vi "Send FindInstruments.vi"(7 "Message Priority (Normal)":T3=enum."Normal", 8 "error in (no error)":errorcluster, 10 "InstrumentData":T1, 11 "Message Enqueuer":refnum<class "Message Enqueuer.lvclass">) -> (0 "error out":errorcluster, 3 "Message Enqueuer out":refnum<class "Message Enqueuer.lvclass">)   [LabVIEW 2023, in "ZWO_ASI.lvlib" / "FindInstruments Msg.lvclass"]
doc: "This VI sends the message to an actor."
uses:
  FindInstruments Msg.lvclass
  FindInstruments Msg.lvclass/FindInstruments Msg.ctl
  <vilib>/ActorFramework/Message Enqueuer/Message Enqueuer.lvclass
  Applications/National Instruments/LabVIEW 2023 64-bit/vi.lib/ActorFramework/Message/Message.lvclass
  Users/alexandrosspiliotis/Documents/LV_DAQ_Project/ConcreteClasses/ConcreteInstrumentClasses/CameraClasses/ZWO_ASI_LV/ZWO_ASI Messages/FindInstruments Msg/FindInstruments Msg.lvclass
  <vilib>/ActorFramework/Message Enqueuer/Message Priority.ctl
  typedefs/instrumentType.ctl
  typedefs/typedefs.lvlib
  typedefs/InstrumentData.ctl
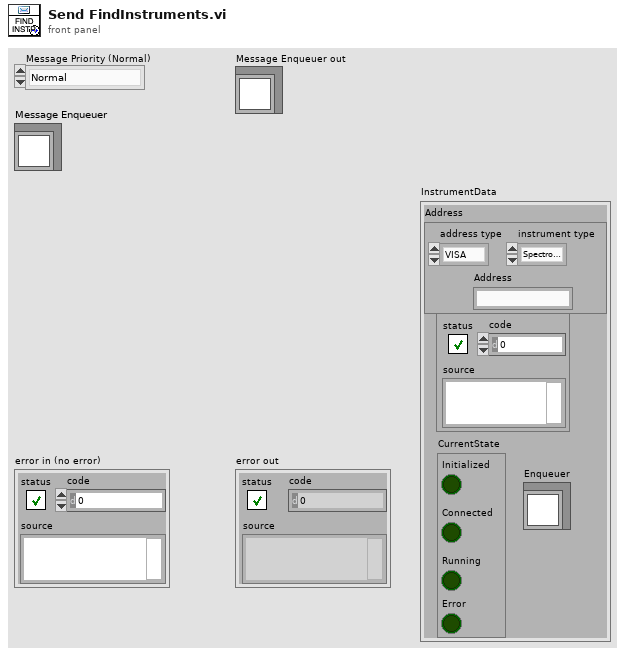
[diagram p1: front panel]
types:
  T1 = typedef "typedefs.lvlib/InstrumentData.ctl" = cluster{"Instr Error":errorcluster, "Address":cluster{"address type":enum16{"VISA", "Index"}, "Address":string, "instrument type":T2}, "CurrentState":cluster{"Initialized":bool, "Connected":bool, "Running":bool, "Error":bool}, "Enqueuer":refnum<class "Message Enqueuer.lvclass">}
  T2 = typedef "typedefs.lvlib/instrumentType.ctl" = enum16{"Spectrometer", "Camera", "Stepper"}
  T3 = typedef "Actor Framework.lvlib/Message Enqueuer.lvclass/Message Priority.ctl" = enum16{"Low", "Normal", "High"}
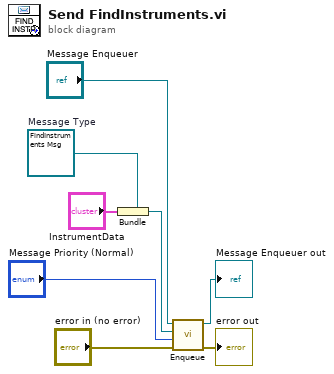
[diagram p0: block diagram]
diagram:
  w5 = refnum<class "FindInstruments Msg.lvclass"> refnum  # Message Type
  n1 = Bundle(cluster=w5, "InstrumentData") -> (w4:refnum<class "FindInstruments Msg.lvclass">)
  n2 = call <vilib>:"Enqueue.vi"("error in (no error)"="error in (no error)", "Message Priority (Normal)"="Message Priority (Normal)", "Message"=w4, "Message Enqueuer in"="Message Enqueuer") -> ("error out"=→"error out":errorcluster, "Message Enqueuer out"=→"Message Enqueuer out":refnum<class "Message Enqueuer.lvclass">)  [unwired: 6 in]
